vi "sbRIO-9651 SPI Simulation.vi"() -> ()   [LabVIEW 2015]
uses:
  Shared Files/SPI Simulation/Controls/Timing Characteristics.ctl
  Shared Files/SPI Simulation/Controls/Digital Data.ctl
  <vilib>/rvi/DesktopExecutionNode/Execution/niFpgaDEN_Execute.vi
  <vilib>/rvi/DesktopExecutionNode/DesktopExecutionNode.xnode
panel:
  in  "SPI Engine Clock Rate (MHz)":i32=120
  in  "SPI Engine Clock Divisor":u8=42
  in  "Transfer Length (bits)":u8=32
  in  "Sample Rate (S/s)":u32=100000 format="%.0p"
  out "Data To Slave":u64 format="%b"
  out "Timing Characteristics":T1 {"tCL (ns)" format="%#_4g"; "tCH (ns)" format="%#_4g"; "tCP (ns)" format="%#_4g"; "tCSS (ns)" format="%#_4g"; "tCSH (ns)" format="%#_4g"; "tCSW (ns)" format="%#_4g"; "Actual Sample Rate (Hz)" format="%_4p"; "SCLK Frequency (Hz)" format="%#.2p"}
  in  "Pause":bool
  out "Digital Data":digitalwaveform(graph)
  in  "Data To Write":u64
  in  "Stop":bool
  # "Operating Instructions\n1. For this VI to work, the FPGA must be in Simulation Mode.\n2. Run the VI and change the 'SPI PHY Settings' and 'Data To Slave' controls to change the SPI Output.\n3. While changing the settings, view the timing characteristics of the signal on the right side of the graph."
  # "Typical Timing Diagram"
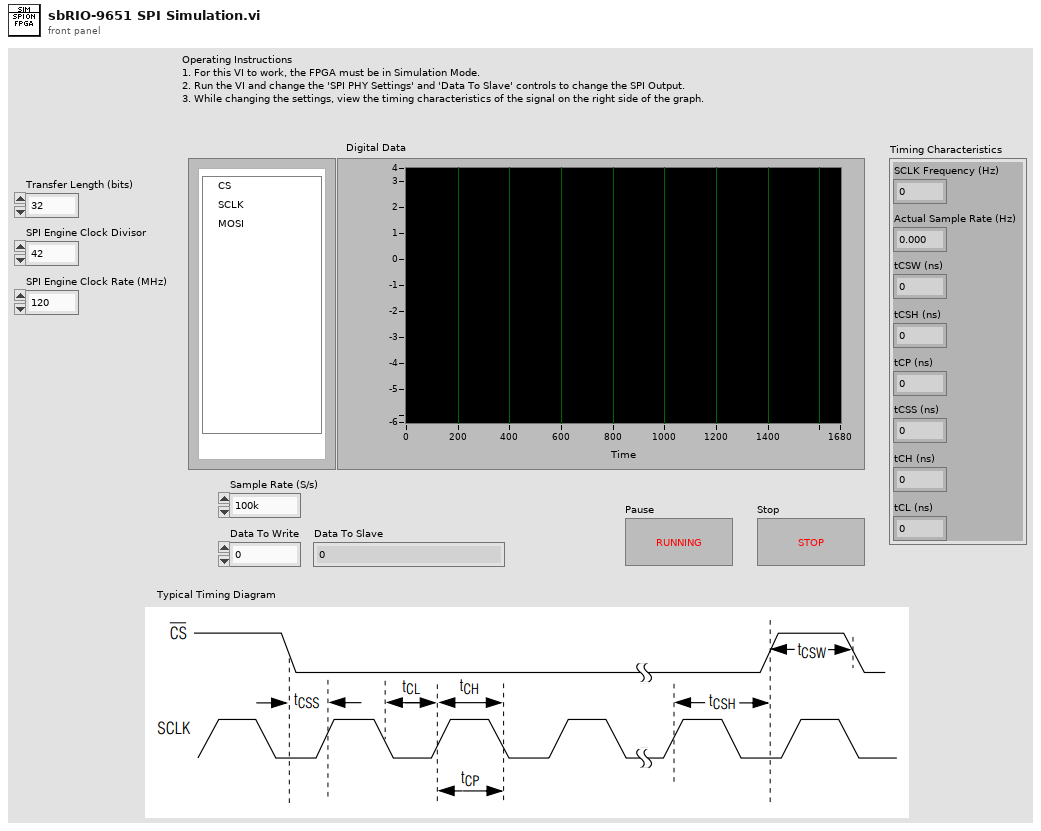
[diagram p1: front panel]
types:
  T1 = typedef "Timing Characteristics.ctl" = cluster{"SCLK Frequency (Hz)":dbl, "Actual Sample Rate (Hz)":dbl, "tCSW (ns)":dbl, "tCSH (ns)":dbl, "tCSS (ns)":dbl, "tCP (ns)":dbl, "tCH (ns)":dbl, "tCL (ns)":dbl}
  T2 = cluster{"Divide Value":u8, "Transfer Length (bits)":u8, "CS Asserted Polarity":bool, "Clock Polarity (CPOL)":bool, "Clock Phase (CPHA)":bool, "Lengthen MISO Setup":bool, "Direction Change Bit":u8, "MOSI Starts as Output":bool, "Tristatable MOSI":bool}
  T3 = typedef "Digital Data.ctl" = cluster{"CS":bool, "SCLK":bool, "MOSI":bool}
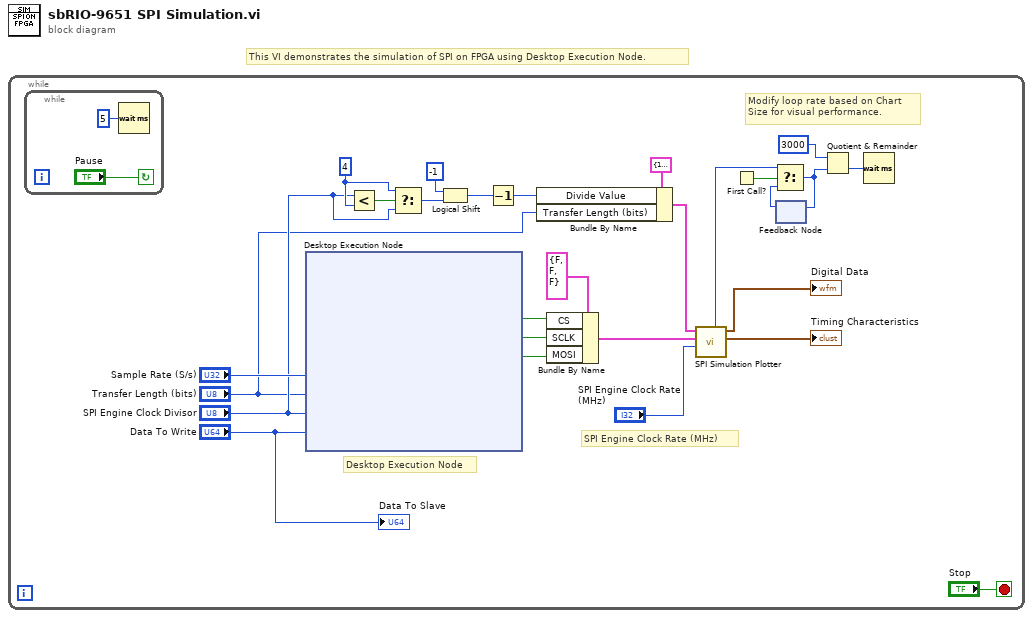
[diagram p0: block diagram]
diagram:
  # "This VI demonstrates the simulation of SPI on FPGA using Desktop Execution Node."
  n1 = while {
    stop <- "Stop" stop-if-true
    w9 = u8 4 ("y")
    # "Desktop Execution Node"
    # "SPI Engine Clock Rate (MHz)"
    # "Modify loop rate based on Chart\nSize for visual performance."
    n2 = while {
      stop <- "Pause" continue-if-true
      n3 = Wait (ms)(milliseconds to wait=u32 5) -> ()  [unwired: 1 out]
    }
    n4 = xnode "Desktop Execution Node"("Sample Rate (S/s)"="Sample Rate (S/s)", "Transfer Length (bits)"="Transfer Length (bits)", "SPI Engine Clock Divisor"="SPI Engine Clock Divisor", "Data To Write"="Data To Write") -> ("CS"=w16:bool, "SCLK"=w15:bool, "MOSI"=w14:bool)  [unwired: 1 in, 1 out]
    n5 = Less?(x="SPI Engine Clock Divisor", y=w9) -> (x < y?=w10:bool)
    n6 = Select(t=w9, s=w10, f="SPI Engine Clock Divisor") -> (s? t:f=w8:u8)
    n7 = Logical Shift(y=i16 -1 ("n"), x=w8) -> (x << y=w6:u8)
    n8 = Decrement(x=w6) -> (x-1=w5:u8)
    n9 = Bundle By Name(cluster=T2 {"Divide Value"=10, "Transfer Length (bits)"=24, "CS Asserted Polarity"=FALSE, "Clock Polarity (CPOL)"=FALSE, "Clock Phase (CPHA)"=FALSE, "Lengthen MISO Setup"=FALSE, "Direction Change Bit"=0, "MOSI Starts as Output"=FALSE, "Tristatable MOSI"=FALSE} ("SPI PHY Settings"), "Divide Value"=w5, "Transfer Length (bits)"="Transfer Length (bits)") -> (w3:T2)
    n10 = Bundle By Name(cluster=T3 {"CS"=FALSE, "SCLK"=FALSE, "MOSI"=FALSE}, "CS"=w16, "SCLK"=w15, "MOSI"=w14) -> (w20:T3)
    n11 = call "SPI Simulation Plotter.vi"("Engine Clock Rate (MHz)"="SPI Engine Clock Rate (MHz)", "SPI Signals"=w20, "SPI PHY Settings"=w3) -> ("Timing Characteristics"=→"Timing Characteristics":T1, "Digital Data"=→"Digital Data":digitalwaveform, "Chart Size"=w19:i32)  [unwired: 6 in]
    n12 = First Call?() -> (First Call?: T/F=w25:bool)
    n13 = feedback #1() -> (w24:i32)  [unwired: 1 in]
    n14 = Select(t=w19, s=w25, f=w24) -> (s? t:f=w23:i32)
    n15 = feedback-in #1(w23) -> ()
    n16 = Quotient & Remainder(x=u32 3000 ("ms per Command"), y=w23) -> (floor(x/y)=w21:u32)  [unwired: 1 out]
    n17 = Wait (ms)(milliseconds to wait=w21) -> ()  [unwired: 1 out]
    "Data To Slave" <- "Data To Write"
  }
